vi "csmdoc_import_VI_description.vi"(6 "Show FP":bool, 7 "LANG ID":string="CＮ", 8 "error in (no error)":errorcluster, 9 "NOTE-Map":variant, 10 "String":string, 11 "Path":path) -> (0 "error out":errorcluster)   [LabVIEW 2017, in "csmdoc.lvlib"]
doc: "-- <b>Controls</b> --\n- <b>NOTE-Map</b>:\n- <b>string</b>:\n- <b>Path</b>:"
uses:
  csmdoc.lvlib
  _Shared/CSM Shared.lvlib
panel:
  out "Array 2":bool[](array[boolean])
  out "Variant":variant
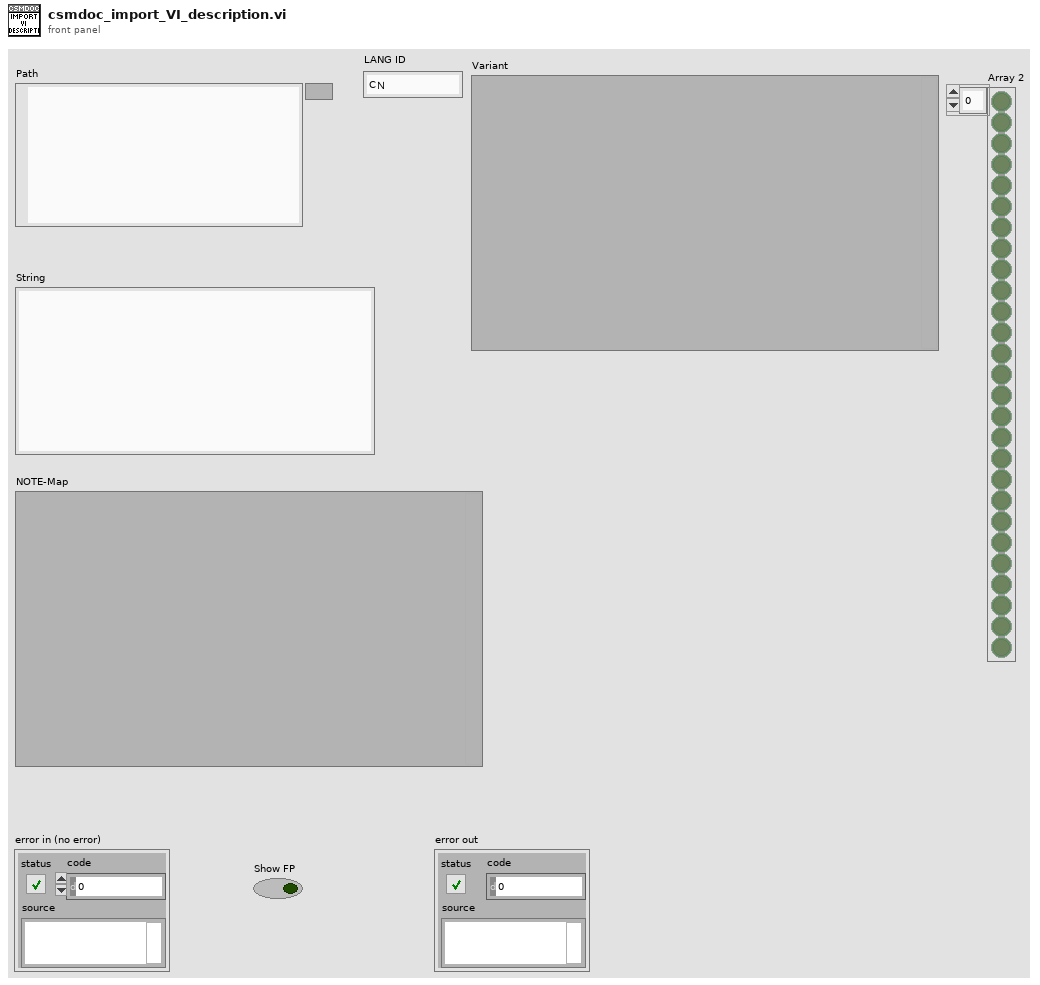
[diagram p1: front panel]
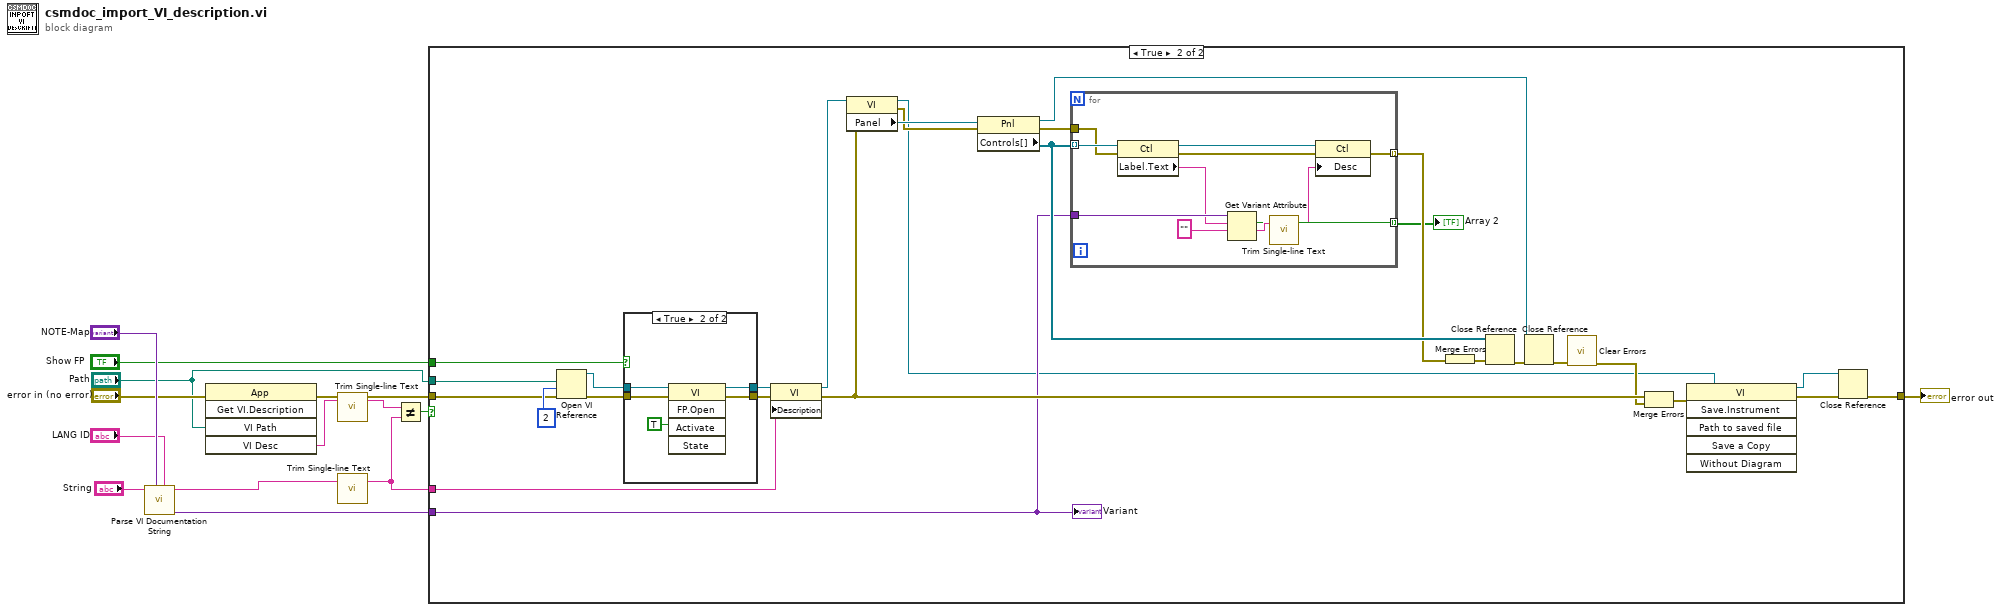
[diagram p0: block diagram]
diagram:
  n1 = call "Parse VI Documentation String.vi"("LANG ID"="LANG ID", "NOTE-Map"="NOTE-Map", "Documentation"="String") -> ("Ctrl-Doc Map"=w13:variant, "Documentation (Dup)"=w10:string)  [unwired: 3 in, 4 out]
  n2 = invoke class="App" method="Get VI.Description"(error in="error in (no error)", "VI Path"="Path") -> (error out=w11:errorcluster, "VI Desc"=w2:string)  [unwired: 3 in, 3 out]
  n3 = call "Trim Single-line Text.vi"("single-line text"=w2) -> ("trimed text"=w8:string)  [unwired: 2 in]
  n4 = call "Trim Single-line Text.vi"("single-line text"=w10) -> ("trimed text"=w7:string)  [unwired: 2 in]
  n5 = Not Equal?(x=w8, y=w7) -> (x != y?=w9:bool)
  n6 = case shown="True" w9 {
    tunnel: w13 -> [_ w30]
    tunnel: w11 -> [w15 w20]
    tunnel: w7 -> [_ w29]
    tunnel: [w15 w17] -> w4
    tunnel: "Show FP" -> [_ w24]
    tunnel: "Path" -> [_ w16]
    frame False {
    }
    frame True {
      n7 = Open VI Reference(vi path=w16, options=2, error in (no error)=w20) -> (vi reference=w21:refnum<vi>, error out=w22:errorcluster)  [unwired: 3 in]
      n8 = case shown="True" w24 {
        tunnel: w22 -> [w44 w49]
        tunnel: w21 -> [w45 w48]
        tunnel: [w44 w47] -> w26
        tunnel: [w45 w46] -> w25
        frame False {
        }
        frame True {
          n9 = invoke class="VI" method="FP.Open"(reference=w48, error in=w49, "Activate"=TRUE ("Activate?")) -> (reference out=w46:refnum<vi>, error out=w47:errorcluster)  [unwired: 2 in, 3 out]
        }
      }
      n10 = property class="VI"(reference=w25, error in=w26, "Description"=w29) -> (reference out=w43:refnum<vi>, error out=w34:errorcluster)
      n11 = property class="VI"(reference=w43, error in=w34) -> (reference out=w27:refnum<vi>, error out=w41:errorcluster, "Panel"=w42:refnum<vi>)
      n12 = property class="Pnl"(reference=w42, error in=w41) -> (reference out=w35:refnum<vi>, error out=w38:errorcluster, "Controls[]"=w40:refnum<vi>[])
      n13 = for {
        tunnel: w40 -> [w61] mode=indexing
        tunnel: w38 -> [w60]
        tunnel: [w57] -> w37 mode=indexing
        tunnel: w30 -> [w56]
        tunnel: [w52] -> w31 mode=indexing
        n14 = property class="Ctl"(reference=w61, error in=w60) -> (reference out=w59:refnum<vi>, error out=w58:errorcluster, "Label.Text"=w55:string)
        n15 = Get Variant Attribute(Variant=w56, name=w55, default value (empty Variant)="" ("regular expression")) -> (found=w52:bool, value=w53:string)  [unwired: 1 in, 2 out]
        n16 = call "Trim Single-line Text.vi"("single-line text"=w53) -> ("trimed text"=w51:string)  [unwired: 2 in]
        n17 = property class="Ctl"(reference=w59, error in=w58, "Desc"=w51) -> (error out=w57:errorcluster)  [unwired: 1 out]
      }
      "Array 2" <- w31
      n18 = Merge Errors(w37) -> (w36:errorcluster)
      n19 = Close Reference(reference=w40, error in (no error)=w36) -> (error out=w39:errorcluster)
      n20 = Close Reference(reference=w35, error in (no error)=w39) -> (error out=w33:errorcluster)
      n21 = call <vilib>:"Clear Errors.vi"("error in (no error)"=w33) -> ("error out"=w32:errorcluster)  [unwired: 5 in, 1 out]
      n22 = Merge Errors(w34, w32) -> (w28:errorcluster)
      n23 = invoke class="VI" method="Save.Instrument"(reference=w27, error in=w28) -> (reference out=w18:refnum<vi>, error out=w19:errorcluster)  [unwired: 4 in, 4 out]
      n24 = Close Reference(reference=w18, error in (no error)=w19) -> (error out=w17:errorcluster)
      "Variant" <- w30
    }
  }
  "error out" <- w4
